vi "setResponseFIFO.vi"(10 "ReadU32FIFO":refnum<class "IReadU32FIFO.lvclass">, 11 "RTHealthAndStatus in":refnum<class "RTHealthAndStatus.lvclass">) -> (3 "RTHealthAndStatus out":refnum<class "RTHealthAndStatus.lvclass">)   [LabVIEW 2016, in "RTHealthAndStatus.lvlib" / "RTHealthAndStatus.lvclass"]
uses:
  RTHealthAndStatus.lvclass
  Common_RT_FPGA/IReadU32FIFO/IReadU32FIFO.lvclass
  RTHealthAndStatus.lvclass/RTHealthAndStatus.ctl
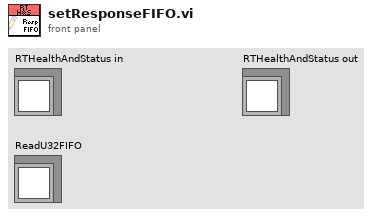
[diagram p1: front panel]
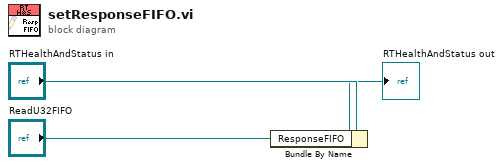
[diagram p0: block diagram]
diagram:
  n1 = Bundle By Name(cluster="RTHealthAndStatus in", "ResponseFIFO"="ReadU32FIFO") -> (→"RTHealthAndStatus out":refnum<class "RTHealthAndStatus.lvclass">)
